vi "Tree Control - Get Route Specification.vi"(8 "error in (no error)":errorcluster, 11 "tree refnum":refnum<vi>) -> (0 "error out":errorcluster, 2 "route specification":string, 3 "tree refnum out":refnum<vi>)   [LabVIEW 2023, in "SwitchExecController.lvlib"]
uses:
  SwitchExecController.lvlib
  <vilib>/Utility/error.llb/Trim Whitespace One-Sided.vi
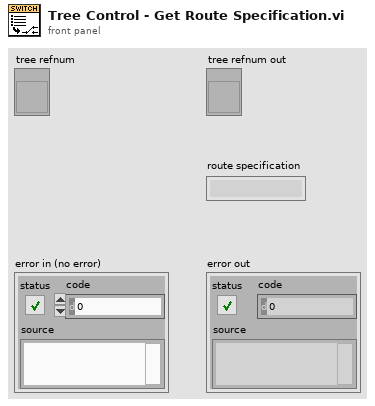
[diagram p1: front panel]
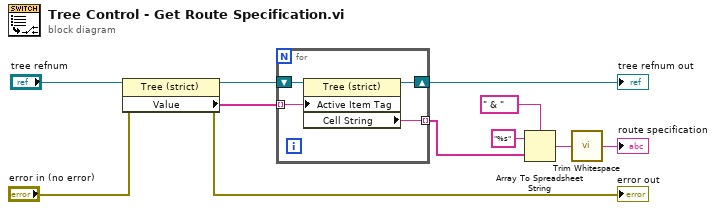
[diagram p0: block diagram]
diagram:
  n1 = property on="Property Node" class="Tree (strict)"(reference="tree refnum", error in="error in (no error)") -> (reference out=w7:refnum<vi>, error out=→"error out":errorcluster, "Value"=w2:string[])
  n2 = for {
    shift-right: [w14] -> w3
    shift-left: w7 -> [w15]
    tunnel: w2 -> [w13] mode=indexing
    tunnel: [w12] -> w1 mode=indexing
    n3 = property class="Tree (strict)"(reference=w15, "Active Item Tag"=w13) -> (reference out=w14:refnum<vi>, "Cell String"=w12:string)  [unwired: 1 in, 1 out]
  }
  "tree refnum out" <- w3
  n4 = Array To Spreadsheet String(delimiter (Tab)=" & ", array=w1, 3:"%s" ("format string")) -> (spreadsheet string=w5:string)
  n5 = call <vilib>:"Trim Whitespace.vi"("string"=w5) -> ("trimmed string"=→"route specification":string)  [unwired: 1 in]
